vi "TestMain.vi"(8 "error in":errorcluster, 11 "Test Folder Path":path) -> (0 "error out":errorcluster, 3 "Array":T1[](array[typedef]))   [LabVIEW 2019]
uses:
  TestResults.ctl
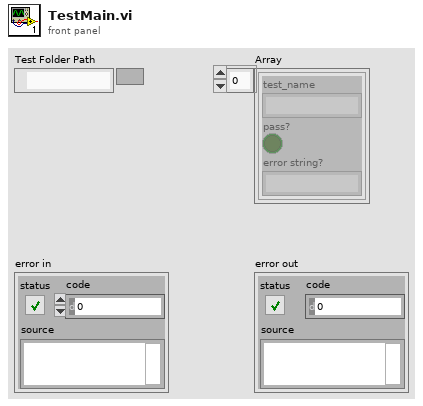
[diagram p1: front panel]
types:
  T1 = typedef "TestResults.ctl" = cluster{"test_name":string, "pass?":bool, "error string?":string}
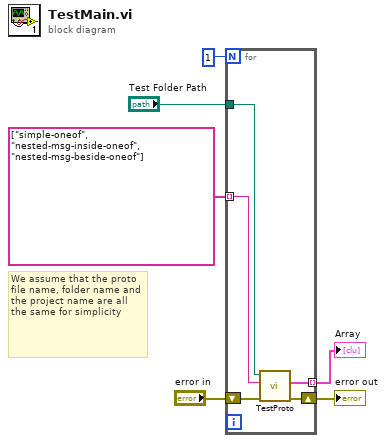
[diagram p0: block diagram]
diagram:
  # "We assume that the proto file name, folder name and the project name are all the same for simplicity"
  n1 = for {
    N: 1 -> [_]
    tunnel: string[] ["simple-oneof", "nested-msg-inside-oneof", "nested-msg-beside-oneof"] -> [w8] mode=indexing
    tunnel: "Test Folder Path" -> [w11]
    shift-right: [w9] -> w2
    shift-left: "error in" -> [w10]
    tunnel: [w7] -> w3 mode=indexing
    n2 = call "TestProto.vi"("error in"=w10, "test name"=w8, "project folder"=w11) -> ("error out"=w9:errorcluster, "test result"=w7:T1)  [unwired: 7 in]
  }
  "Array" <- w3
  "error out" <- w2
